vi "cnts2mmThorLabs.vi"(11 "XYX cmd [enc cnts]":i32) -> (3 "XYZ cmd [mm]":dbl)   [LabVIEW 2016]
panel:
  # ">>>"
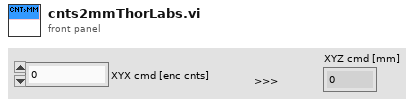
[diagram p1: front panel]
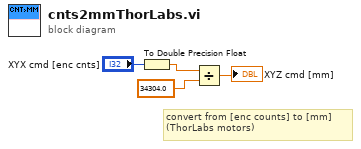
[diagram p0: block diagram]
diagram:
  # "convert from [enc counts] to [mm]\n(ThorLabs motors)"
  n1 = To Double Precision Float(number="XYX cmd [enc cnts]") -> (double precision float=w1:dbl)
  n2 = Divide(x=w1, y=34304.0) -> (x/y=→"XYZ cmd [mm]":dbl)
